vi "example_06_cursors.vi"() -> ()   [LabVIEW 2015, in "lv-graph.lvlib"]
doc: "This example provides a showcase of the cursor functions that try to simplify basic workflows for interacting with cursors as in creating them, configuring them and moving them."
uses:
  public/_controls/configuration_cursor.ctl
  public/advanced/build_graph-single_axis.vi
  lv-graph.lvlib
panel:
  in  "index":i32
  in  "move_cursor":bool
  in  "active_cursor":u32
  in  "copy_cursor":bool
  in  "cursor_configuration":T1={"active_cursor"=0, "allow_drag"=TRUE, "color"=6618880, "mode"=1, "name"="cursor", "name_visible"=TRUE, "cursor_plot"=0, "point_style"=3, "selection_color"=0, "style"=0, "line_style"=0, "line_width"=0, "plot_area"=0, "visible"=TRUE, "watch_all_plots"=TRUE, "x_scale"=0, "y_scale"=0}
  in  "set_cursor":bool
  in  "number_of_points_to_generate":i32=1000
  in  "stop":bool
  out "graph":T2(graph)
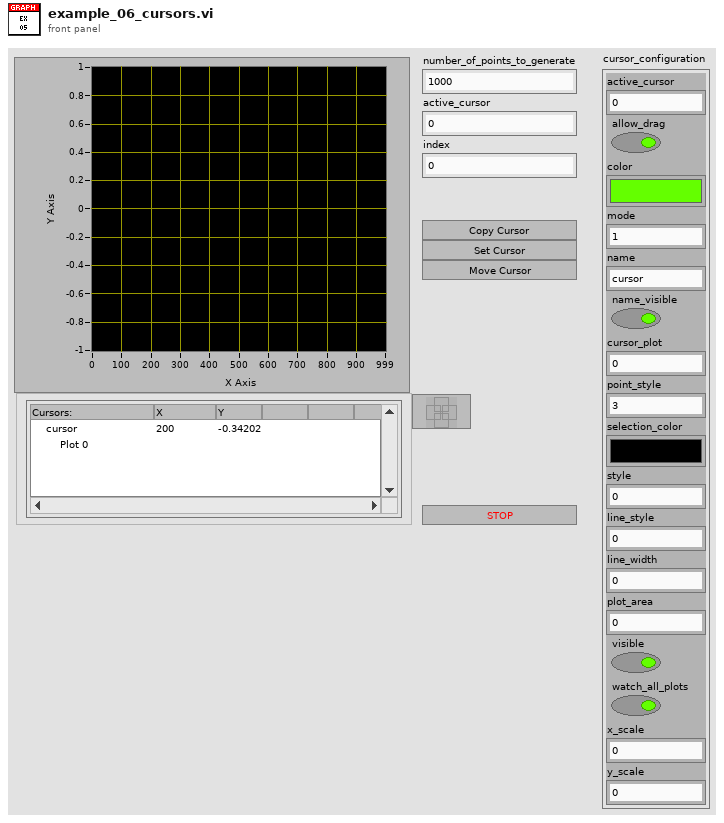
[diagram p1: front panel]
types:
  T1 = typedef "lv-graph.lvlib/configuration_cursor.ctl" = cluster{"active_cursor":u32, "allow_drag":bool, "color":u32, "mode":u32, "name":string, "name_visible":bool, "cursor_plot":i32, "point_style":u8, "selection_color":u32, "style":u8, "line_style":u8, "line_width":u8, "plot_area":i32, "visible":bool, "watch_all_plots":bool, "x_scale":u32, "y_scale":u32}
  T2 = cluster{"Time [] out":dbl[], "Data[][] out":dbl[]}[]
  T3 = cluster{"x_scale_maximum":dbl, "x_scale_minimum":dbl, "y_scale_maximum":dbl, "y_scale_minimum":dbl}
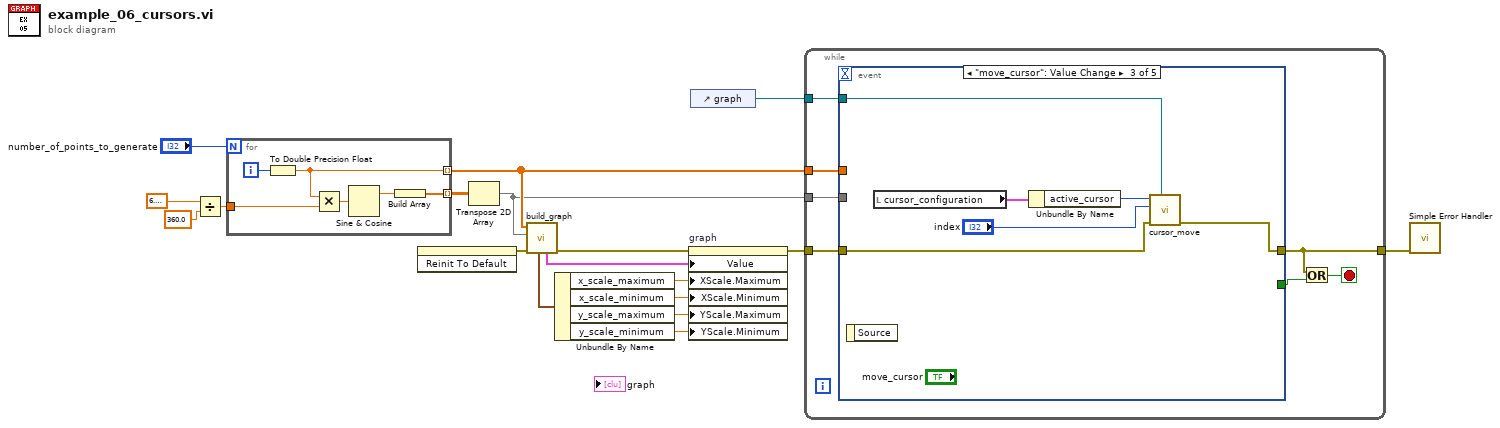
[diagram p0: block diagram]
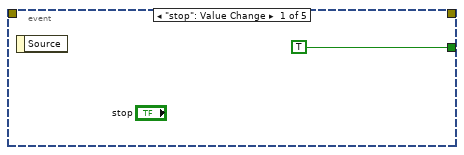
[diagram p2: hidden frame]
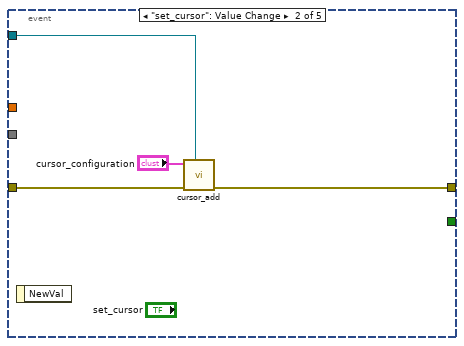
[diagram p3: hidden frame]
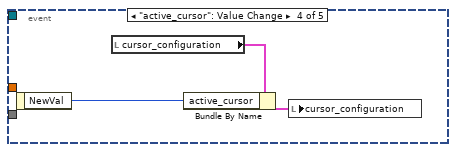
[diagram p4: hidden frame]
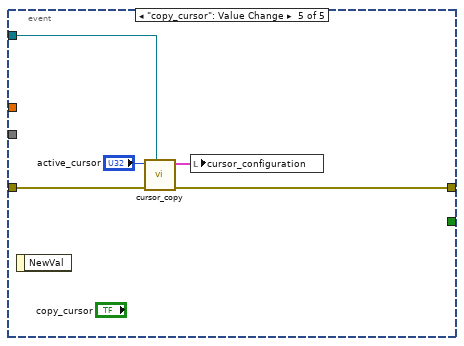
[diagram p5: hidden frame]
diagram:
  n1 = Divide(x=6.283185307179586, y=360.0) -> (x/y=w4:dbl)
  n2 = for {
    N: "number_of_points_to_generate" -> [_]
    tunnel: [w20] -> w11 mode=indexing
    tunnel: [w22] -> w2 mode=indexing
    tunnel: w4 -> [w19]
    i -> [w21]
    n3 = To Double Precision Float(number=w21) -> (double precision float=w22:dbl)
    n4 = Multiply(x=w22, y=w19) -> (x*y=w23:dbl)
    n5 = Sine & Cosine(0:w23) -> (1:w24:dbl)  [unwired: 1 out]
    n6 = Build Array(w24) -> (w20:dbl[])
  }
  n7 = invoke on="stop" class="Bool" method="Reinit To Default"() -> (error out=w3:errorcluster)  [unwired: 3 in, 2 out]
  n8 = Transpose 2D Array(2D array=w11) -> (transposed array=w1:dbl[][])
  n9 = call-poly "build_graph.vi"("error in (no error)"=w3, "y_axis"=w1, "x_axis"=w2) -> ("error out"=w18:errorcluster, "graph_data"=w12:cluster{dbl[], dbl[]}[], "scale_ranges"=w13:T3)  [unwired: 6 in]
  n10 = Unbundle By Name(w13) -> ("x_scale_maximum"=w16:dbl, "x_scale_minimum"=w17:dbl, "y_scale_maximum"=w15:dbl, "y_scale_minimum"=w14:dbl)
  n11 = property on="graph" class="XYGraph (strict)"(error in=w18, "Value"=w12, "XScale.Maximum"=w16, "XScale.Minimum"=w17, "YScale.Maximum"=w15, "YScale.Minimum"=w14) -> (error out=w9:errorcluster)  [unwired: 1 in, 1 out]
  n12 = control-ref of="graph"() -> (w8:refnum<vi>)
  n13 = while {
    tunnel: w9 -> [w31]
    tunnel: w8 -> [w28]
    tunnel: [w27] -> w7
    tunnel: w2 -> [w26]
    tunnel: w1 -> [w25]
    stop <- w29 stop-if-true
    n14 = event shown="[2] \"move_cursor\": Value Change" {
      selector: _ -> [_ _ _ _ _]
      dyn-events: _ -> [_ _ _ _ _]
      timeout: _ -> [_ _ _ _ _]
      tunnel: [TRUE _ _ _ _] -> w30
      tunnel: w31 -> [_ w36 w41 _ w50]
      tunnel: w28 -> [_ w35 w42 _ w49]
      tunnel: [_ w33 w40 _ w48] -> w27
      tunnel: w26 -> [_ _ _ _ _]
      tunnel: w25 -> [_ _ _ _ _]
      event "stop": Value Change {
        n15 = event-data() -> ()  [unwired: 1 in, 1 out]
      }
      event "set_cursor": Value Change {
        n16 = event-data() -> ()  [unwired: 1 in, 1 out]
        n17 = call "cursor_add.vi"("xy_graph_reference"=w35, "error in (no error)"=w36, "cursor_configuration"="cursor_configuration") -> ("error out"=w33:errorcluster)  [unwired: 8 in]
      }
      event "move_cursor": Value Change {
        n18 = event-data() -> ()  [unwired: 1 in, 1 out]
        n19 = local read "cursor_configuration"() -> (w39:T1)
        n20 = Unbundle By Name(w39) -> ("active_cursor"=w38:u32)
        n21 = call "cursor_move.vi"("xy_graph_reference"=w42, "error in (no error)"=w41, "cursor_index"="index", "active_cursor"=w38) -> ("error out"=w40:errorcluster)  [unwired: 7 in]
      }
      event "active_cursor": Value Change {
        n22 = event-data() -> ("NewVal"=w43:u32)  [unwired: 1 in]
        n23 = local read "cursor_configuration"() -> (w45:T1)
        n24 = Bundle By Name(cluster=w45, "active_cursor"=w43) -> (w44:T1)
        n25 = local write "cursor_configuration"(w44) -> ()
      }
      event "copy_cursor": Value Change {
        n26 = event-data() -> ()  [unwired: 1 in, 1 out]
        n27 = call "cursor_copy.vi"("xy_graph_reference"=w49, "error in (no error)"=w50, "active_curosr"="active_cursor") -> ("error out"=w48:errorcluster, "cursor_configuration"=w47:T1)  [unwired: 7 in]
        n28 = local write "cursor_configuration"(w47) -> ()
      }
    }
    n29 = Or(x=w27, y=w30) -> (x .or. y?=w29:bool)
  }
  n30 = call <vilib>:"Simple Error Handler.vi"("error in (no error)"=w7) -> ()  [unwired: 4 in, 5 out]
